vi "Query Max Voltage Level.vi"(8 "error in (no error)":errorcluster, 9 "current limit (0.0 Amps)":dbl[unit] format="%^.2e", 10 "channel name (\"CHANNEL1\")":string="CHANNEL1", 11 "CS++DCPwr in":refnum<class "CS++DCPwr.lvclass">) -> (0 "error out":errorcluster, 2 "max voltage level":dbl[unit] format="%^.2e", 3 "CS++DCPwr out":refnum<class "CS++DCPwr.lvclass">)   [LabVIEW 2016, in "CS++DCPwr.lvlib" / "CS++DCPwr.lvclass"]
doc: "This VI returns the maximum programmable voltage level that the power supply accepts for a particular current limit on a channel for the output range to which the power supply is currently configured."
uses:
  CS++DCPwr.lvclass
  CSPP_Core/Classes/CS++ProcessVariables/ProcessVariable/PV.lvclass
  PV-Enum.ctl
  CSPP_Core/Classes/CS++ProcessVariables/ProcessVariable/PV.lvclass/PV.ctl
  CS++DCPwr.lvclass/CS++DCPwr.ctl
  CSPP_Core/Classes/CS++ProcessVariables/ProcessVariable/Write Data.vi
  CSPP_Core/Classes/CS++ProcessVariables/ProcessVariable/Write Timestamp.vi
  CSPP_Core/Classes/CS++ProcessVariables/ProcessVariable/Write Quality.vi
  CSPP_Core/Classes/CS++ProcessVariables/ProcessVariable/Write status.vi
  CSPP_Core/Classes/CS++ProcessVariables/PVConnection/PVConnection.lvclass
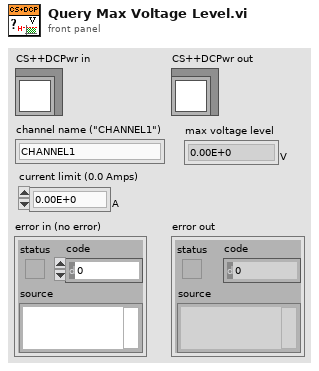
[diagram p1: front panel]
types:
  T1 = typedef "CS++DCPwr.lvlib/CS++DCPwr.lvclass/PV-Enum.ctl" = enum16{"CurrentLimit", "MaxCurrentLimit", "MaxVoltageLevel", "Measure-A", "Measure-V", "OVPLimit", "Range", "TriggerCurrentLimit", "TriggerVoltageLevel", "VoltageLevel", "Behavior", "DesiredOutputState", "RangeType", "TriggerSource", "InState", "OutputEnable", "OVPEnabled"}
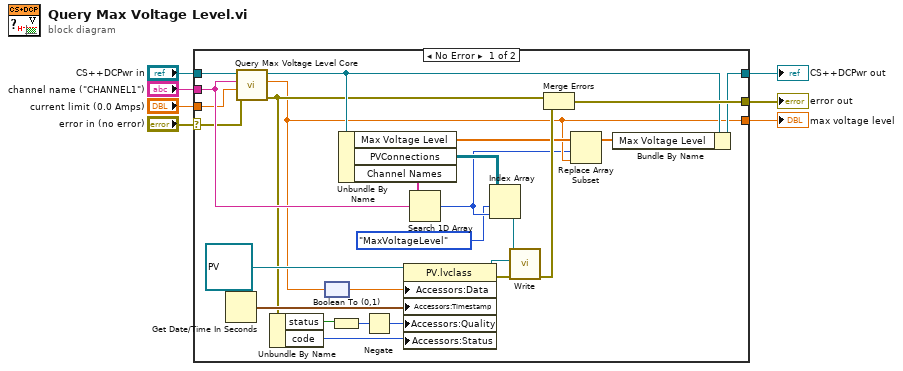
[diagram p0: block diagram]
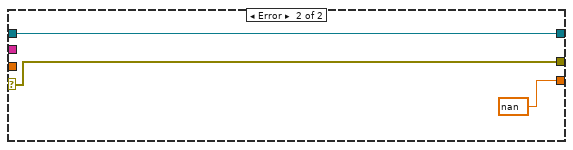
[diagram p2: hidden frame]
diagram:
  n1 = case shown="No Error" "error in (no error)" {
    selector: "error in (no error)" -> [w14 w35]
    tunnel: "CS++DCPwr in" -> [w17 w36]
    tunnel: "current limit (0.0 Amps)" -> [w15 _]
    tunnel: "channel name (\"CHANNEL1\")" -> [w16 _]
    tunnel: [w21 w35] -> w5
    tunnel: [w20 w36] -> w7
    tunnel: [w11 dbl[unit] nan ("max current limit")] -> w6
    frame No Error {
      n2 = Get Date/Time In Seconds() -> (seconds since 1Jan1904=w33:timestamp)
      n3 = call-dynamic "Query Max Voltage Level Core.vi"("error in (no error)"=w14, "current limit (0.0 Amps)"=w15, "channel name (\"CHANNEL1\")"=w16, "CS++DCPwr in"=w17) -> ("error out"=w12:errorcluster, "max voltage level"=w11:dbl[unit], "CS++DCPwr out"=w13:refnum<class "CS++DCPwr.lvclass">)  [unwired: 5 in]
      n4 = Unbundle By Name(w12) -> ("status"=w25:bool, "code"=w23:i32)
      n5 = node(w11) -> (w10:dbl)
      n6 = Boolean To (0,1)(Boolean=w25) -> (0, 1=w24:i16)
      n7 = Unbundle By Name(w13) -> ("Max Voltage Level"=w19:dbl[unit][], "PVConnections"=w28:refnum<class "PVConnection.lvclass">[][], "Channel Names"=w29:string[])
      n8 = Negate(x=w24) -> (-x=w22:i16)
      n9 = property class="PV.lvclass"(reference=refnum<class "PV.lvclass"> refnum ("PV"), "Accessors:Data"=w10, "Accessors:Timestamp"=w33, "Accessors:Quality"=w22, "Accessors:Status"=w23) -> (reference out=w30:refnum<class "PV.lvclass">, error out=w31:errorcluster)  [unwired: 1 in]
      n10 = Search 1D Array(1D array=w29, element=w16) -> (index of element=w9:i32)  [unwired: 1 in]
      n11 = Index Array(array=w28, index (row)=PV-Enum."MaxVoltageLevel" ("PV-Enum"), index (col)=w9) -> (element=w27:refnum<class "PVConnection.lvclass">)
      n12 = call "Write.vi"("error in (no error)"=w31, "PV"=w30, "PVConnection in"=w27) -> ("error out"=w26:errorcluster)  [unwired: 7 in, 1 out]
      n13 = Merge Errors(w12, w26) -> (w21:errorcluster)
      n14 = Replace Array Subset(array=w19, new element=w11, index=w9) -> (w18:dbl[unit][])
      n15 = Bundle By Name(cluster=w13, "Max Voltage Level"=w18) -> (w20:refnum<class "CS++DCPwr.lvclass">)
    }
    frame Error {
    }
  }
  "error out" <- w5
  "CS++DCPwr out" <- w7
  "max voltage level" <- w6
